vi "M0 Hybrid car.vi"(11 "NXT/EV3":T1) -> (3 "EV3 out":T1)   [LabVIEW 2016]
uses:
  <vilib>/NXT/Subs/LVHSConnector.ctl
  <vilib>/NXT/LegoClasses/BrickReference/BrickReference.lvclass
  <vilib>/NXT/Dual Mode Library/Waits/Wait_Num.vi
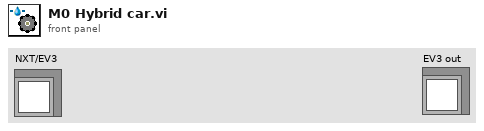
[diagram p1: front panel]
types:
  T1 = typedef "LVHSConnector.ctl" = refnum<class "BrickReference.lvclass">
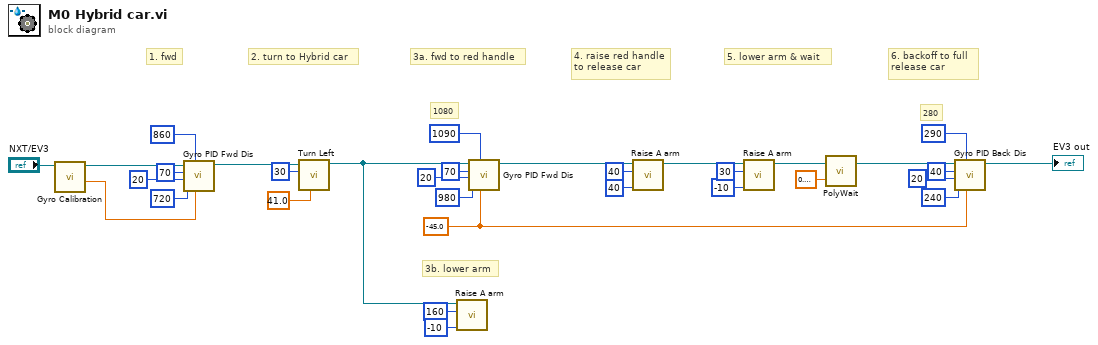
[diagram p0: block diagram]
diagram:
  w5 = sgl -45.0 ("Target angle")
  # "280"
  # "1080"
  # "6. backoff to full\nrelease car"
  # "5. lower arm & wait"
  # "4. raise red handle\nto release car"
  # "3b. lower arm"
  # "3a. fwd to red handle"
  # "2. turn to Hybrid car"
  # "1. fwd"
  n1 = call "Gyro Calibration.vi"("NXT/EV3"="NXT/EV3") -> ("Degrees"=w27:sgl, "NXT/EV3"=w32:T1)  [unwired: 6 in, 1 out]
  n2 = call "Gyro PID Fwd Dis.vi"("Target angle"=w27, "Threshold to stop"=860, "Threshold to slow"=720, "Min. speed"=20, "Max. speed"=70, "EV3 in"=w32) -> ("EV3 out"=w20:T1)  [unwired: 5 in]
  n3 = call "Turn Left.vi"("Turning angle"=sgl 41.0, "Motor B (right)"=i8 30, "EV3 in"=w20) -> ("EV3 out"=w19:T1)  [unwired: 8 in]
  n4 = call "Raise A arm.vi"("Power"=i8 -10, "Rotation"=160, "EV3 in"=w19) -> ()  [unwired: 8 in, 1 out]
  n5 = call "Gyro PID Fwd Dis.vi"("Target angle"=w5, "Threshold to stop"=1090, "Threshold to slow"=980, "Min. speed"=20, "Max. speed"=70, "EV3 in"=w19) -> ("EV3 out"=w15:T1)  [unwired: 5 in]
  n6 = call "Raise A arm.vi"("Power"=i8 40, "Rotation"=40, "EV3 in"=w15) -> ("EV3 out"=w11:T1)  [unwired: 8 in]
  n7 = call "Raise A arm.vi"("Power"=i8 -10, "Rotation"=30, "EV3 in"=w11) -> ("EV3 out"=w10:T1)  [unwired: 8 in]
  n8 = call-poly <vilib>:"PolyWait.vi"("Time (1 sec)"=sgl 0.2, "NXT/EV3"=w10) -> ("NXT/EV3"=w4:T1)  [unwired: 2 in]
  n9 = call "Gyro PID Back Dis.vi"("Target angle"=w5, "Threshold to stop"=290, "Threshold to slow"=240, "Min. speed"=20, "Max. speed"=40, "EV3 in"=w4) -> ("EV3 out"=→"EV3 out":T1)  [unwired: 5 in]
